vi "PROIECT2.vi"() -> ()   [LabVIEW 2021]
panel:
  in  "Radio Buttons":enum32{"FORMULA 1", "FORMULA2"}(radio)
  in  "stop":bool
  in  "x":dbl
  in  "k":dbl(slide) scale=0.0..10.0
  out "Waveform Graph":i32[](graph)
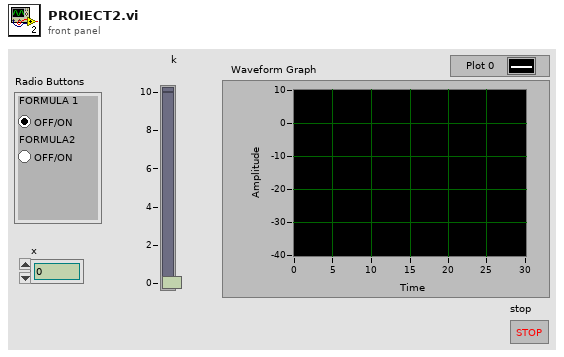
[diagram p1: front panel]
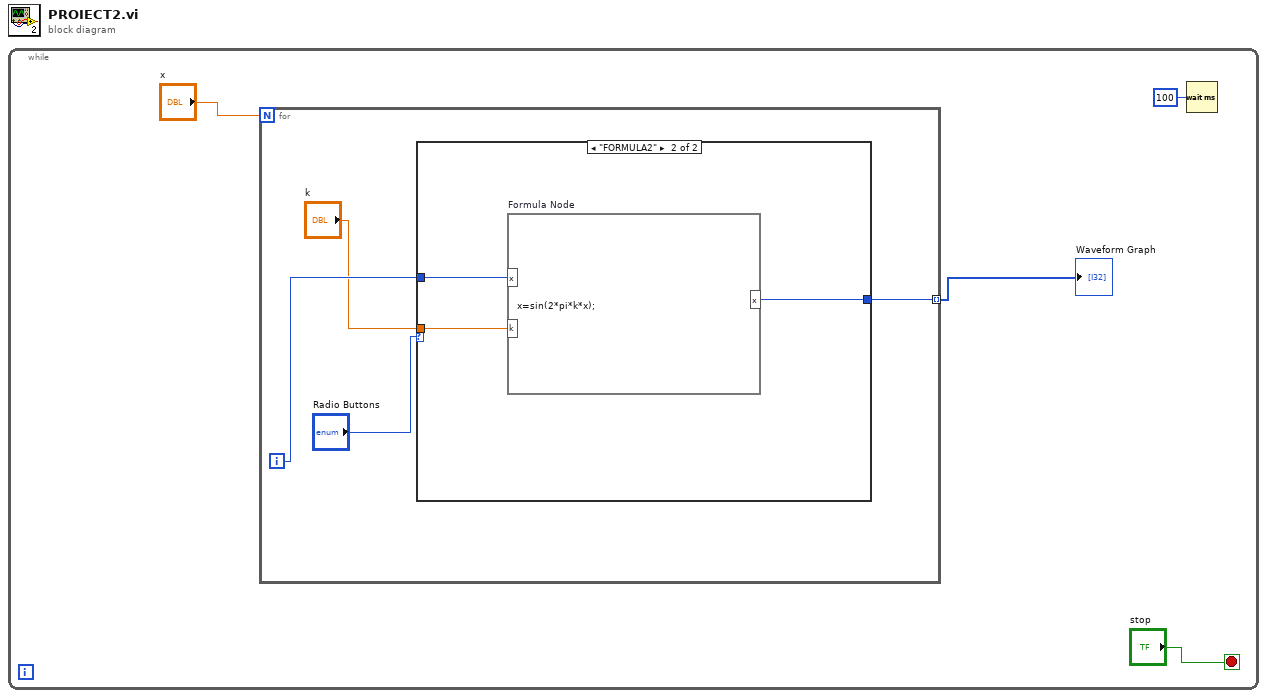
[diagram p0: block diagram]
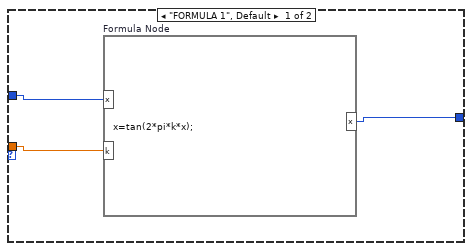
[diagram p2: hidden frame]
diagram:
  n1 = while {
    stop <- "stop" stop-if-true
    n2 = for {
      N: "x" -> [_]
      tunnel: [w7] -> w3 mode=indexing
      i -> [w8]
      n3 = case shown="\"FORMULA2\"" "Radio Buttons" {
        tunnel: w8 -> [w9 w14]
        tunnel: [w11 w13] -> w7
        tunnel: "k" -> [w10 w12]
        frame "FORMULA 1", Default {
          n4 = formula code="x=tan(2*pi*k*x);"("k"=w10, "x"=w9) -> ("x"=w11:i32)
        }
        frame "FORMULA2" {
          n5 = formula code="x=sin(2*pi*k*x);"("k"=w12, "x"=w14) -> ("x"=w13:i32)
        }
      }
    }
    "Waveform Graph" <- w3
    n6 = Wait (ms)(milliseconds to wait=u32 100) -> ()  [unwired: 1 out]
  }
